vi "VI Server_TREE_Header_Color_SET.vi"(6 "Header.Color":u32(colorbox)=16777226, 7 "Label":string, 8 "error in":errorcluster, 9 "Tree.Ref":refnum<vi>, 11 "VI Server.RefsCluster":T1) -> (0 "error out":errorcluster, 1 "Tree.Ref.DUP":refnum<vi>, 3 "VI Server.RefsCluster.DUP":T1)   [LabVIEW 2020]
uses:
  VI Server_TypeDefs/VI Server_RefsCluster.ctl
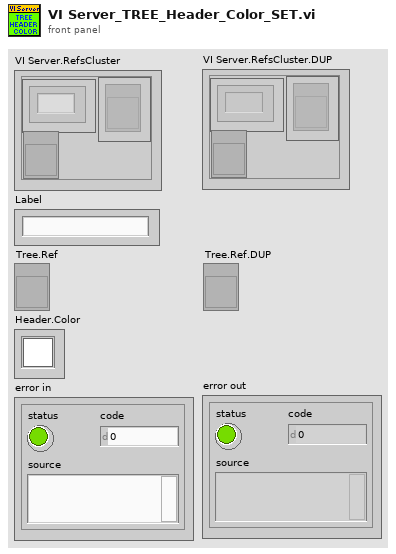
[diagram p1: front panel]
types:
  T1 = typedef "VI Server_RefsCluster.ctl" = cluster{"Labels":string[], "Refs":refnum<vi>[], "VI Ref":refnum<vi>}
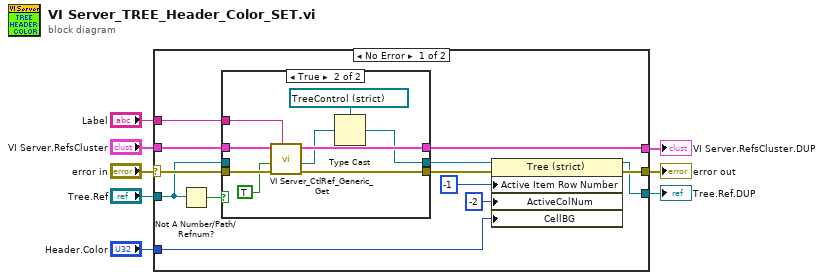
[diagram p0: block diagram]
diagram:
  n1 = case shown="No Error" "error in" {
    selector: "error in" -> [w21 w35]
    tunnel: [w14 w35] -> w7
    tunnel: "VI Server.RefsCluster" -> [w20 w34]
    tunnel: [w19 w34] -> w5
    tunnel: "Label" -> [w18 _]
    tunnel: [w12 _] -> w1
    tunnel: "Tree.Ref" -> [w16 _]
    tunnel: "Header.Color" -> [w11 _]
    frame No Error {
      n2 = Not A Number/Path/Refnum?(number/path/refnum=w16) -> (NaN/Path/Refnum?=w17:bool)
      n3 = case shown="True" w17 {
        tunnel: w21 -> [w24 w33]
        tunnel: w20 -> [w22 w32]
        tunnel: [w22 w31] -> w19
        tunnel: w18 -> [_ w30]
        tunnel: [w23 w28] -> w13
        tunnel: [w24 w27] -> w15
        tunnel: w16 -> [w23 _]
        frame False {
        }
        frame True {
          n4 = call "VI Server_CtlRef_Generic_Get.vi"("Control.Label"=w30, "error in"=w33, "SingleInstance"=TRUE, "VI Server.RefsCluster"=w32) -> ("error out"=w27:errorcluster, "Control.Ref.Generic"=w29:refnum<vi>, "VI Server.RefsCluster.DUP"=w31:T1)  [unwired: 5 in]
          n5 = Type Cast(type=refnum<vi> refnum ("Test.Tree"), x=w29) -> (*(type *) &x=w28:refnum<vi>)
        }
      }
      n6 = property on="Property Node" class="Tree (strict)"(reference=w13, error in=w15, "Active Item Row Number"=-1 ("Row Number\n(-2-all clmns)"), "ActiveColNum"=-2 ("Column Number\n(-2 - whole row)"), "CellBG"=w11) -> (reference out=w12:refnum<vi>, error out=w14:errorcluster)
    }
    frame Error {
    }
  }
  "VI Server.RefsCluster.DUP" <- w5
  "error out" <- w7
  "Tree.Ref.DUP" <- w1
